vi "Pump Start Detector (Kuhnke) old.vi"(6 "Reset":bool, 9 "Period":i32, 10 "Neg Cross":bool, 11 "Pos Cross":bool) -> (3 "Starts":u32)   [LabVIEW 2019]
uses:
  <vilib>/Platform/TimedLoop/XDataNode/timing_clust.ctl
  <vilib>/Platform/TimedLoop/XDataNode/nitl_modes.ctl
  <vilib>/Platform/TimedLoop/XDataNode/wakeup.ctl
  <vilib>/Platform/TimedLoop/XDataNode/XDataNode.xnode
  <vilib>/Platform/TimedLoop/XDataNode/XDNodeRunTimeDep.lvlib
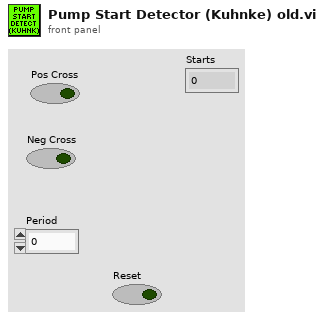
[diagram p1: front panel]
types:
  T1 = typedef "XDNodeRunTimeDep.lvlib/timing_clust.ctl" = cluster{"Expected End [f-1]":u64, "Actual End [f-1]":u64, "Finished Late? [f-1]":bool, "Expected End [i-1]":u64, "Actual End [i-1]":u64, "Finished Late? [i-1]":bool, "Expected Start [i]":u64, "Actual Start [i]":u64, "Expected Start [f]":u64, "Actual Start [f]":u64, "Source Name":string, "Structure Name":string, "Period":i64, "Deadline":i64, "Offset":i64, "Start":i64, "Priority":i32, "Timeout":i32, "Mode":T2, "Wakeup Reason":T3, "Error":errorcluster, "Source Type":string, "Secondary Source Type":string, "Global End Time":u64, "Global Start Time":u64, "Frame Duration":u64, "Iteration Duration":u64, "Assigned CPU":i32, "I/O Scan Engine Mode":u32}
  T2 = typedef "XDNodeRunTimeDep.lvlib/nitl_modes.ctl" = enum32{"No Change", "Process missed periods, maintain original phase", "Discard missed periods, maintain original phase", "Process missed periods, ignore original phase", "Discard missed periods, ignore original phase"}
  T3 = typedef "XDNodeRunTimeDep.lvlib/wakeup.ctl" = enum32{"Normal", "Aborted", "Asynchronous wakeup", "Timing source error", "Timed loop error", "Timeout"}
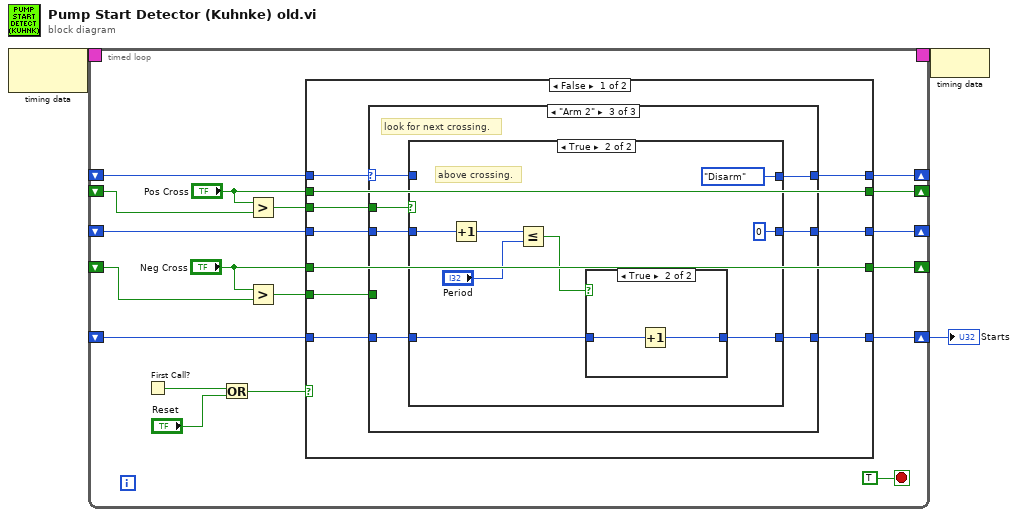
[diagram p0: block diagram]
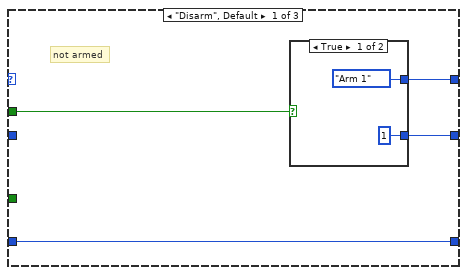
[diagram p2: hidden frame]
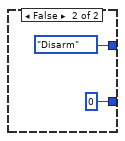
[diagram p3: hidden frame]
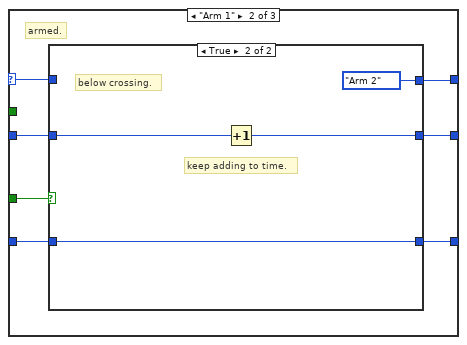
[diagram p4: hidden frame]
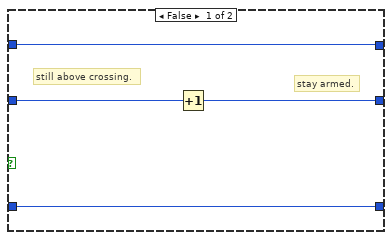
[diagram p5: hidden frame]
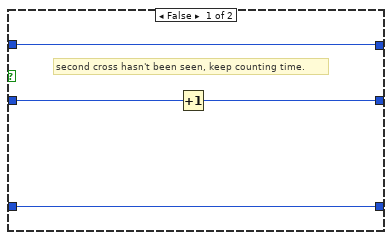
[diagram p6: hidden frame]
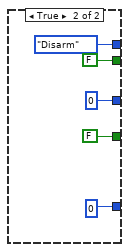
[diagram p8: hidden frame]
diagram:
  n1 = node-c288() -> (w3:T1)  [unwired: 1 in]
  n2 = timed-loop {
    shift-right: [w15] -> w1
    shift-left: _ -> [w16]
    shift-right: [w20] -> _
    shift-left: _ -> [w21]
    shift-right: [w19] -> _
    shift-left: _ -> [w18]
    timing: w3 -> [_]
    timing-out: [_] -> w2
    shift-right: [w12] -> _
    shift-left: _ -> [w10]
    shift-right: [w7] -> _
    shift-left: _ -> [w5]
    stop <- TRUE stop-if-true
    n3 = First Call?() -> (First Call?: T/F=w14:bool)
    n4 = Or(x=w14, y="Reset") -> (x .or. y?=w13:bool)
    n5 = Greater?(x="Pos Cross", y=w10) -> (0:w11:bool)
    n6 = Greater?(x="Neg Cross", y=w5) -> (0:w4:bool)
    n7 = case shown="False" w13 {
      tunnel: w21 -> [w31 _]
      tunnel: [w30 enum16{"Arm 1", "Arm 2", "Disarm"}."Disarm"] -> w20
      tunnel: [w29 0] -> w19
      tunnel: w18 -> [w28 _]
      tunnel: w16 -> [w27 _]
      tunnel: [w26 u32 0] -> w15
      tunnel: "Pos Cross" -> [w25 _]
      tunnel: [w25 FALSE ("Crossing?")] -> w12
      tunnel: w11 -> [w24 _]
      tunnel: "Neg Cross" -> [w23 _]
      tunnel: [w23 FALSE ("Neg Cross")] -> w7
      tunnel: w4 -> [w22 _]
      frame False {
        n8 = case shown="\"Arm 2\"" w31 {
          selector: w31 -> [_ w41 w55]
          tunnel: [w32 w46 w60] -> w30
          tunnel: [w34 w45 w59] -> w29
          tunnel: w28 -> [_ w44 w58]
          tunnel: w24 -> [w33 _ w61]
          tunnel: w27 -> [w35 w43 w57]
          tunnel: [w35 w42 w56] -> w26
          tunnel: w22 -> [_ w40 _]
          frame "Disarm", Default {
            # "not armed"
            n9 = case shown="True" w33 {
              tunnel: [1 0] -> w34
              tunnel: [enum16{"Arm 1", "Arm 2", "Disarm"}."Arm 1" enum16{"Arm 1", "Arm 2", "Disarm"}."Disarm"] -> w32
              frame True {
              }
              frame False {
              }
            }
          }
          frame "Arm 1" {
            # "armed."
            n10 = case shown="True" w40 {
              tunnel: [w47 enum16{"Arm 1", "Arm 2", "Disarm"}."Arm 2"] -> w46
              tunnel: [w49 w51] -> w45
              tunnel: w44 -> [w50 w52]
              tunnel: w43 -> [w48 w54]
              tunnel: [w48 w54] -> w42
              tunnel: w41 -> [w47 _]
              frame False {
                # "stay armed."
                # "still above crossing."
                n11 = Increment(x=w50) -> (x+1=w49:i32)
              }
              frame True {
                # "keep adding to time."
                # "below crossing."
                n12 = Increment(x=w52) -> (x+1=w51:i32)
              }
            }
          }
          frame "Arm 2" {
            # "look for next crossing."
            n13 = case shown="True" w61 {
              tunnel: [w62 enum16{"Arm 1", "Arm 2", "Disarm"}."Disarm"] -> w60
              tunnel: [w64 0] -> w59
              tunnel: w58 -> [w65 w71]
              tunnel: w57 -> [w63 w70]
              tunnel: [w63 w69] -> w56
              tunnel: w55 -> [w62 _]
              frame False {
                # "second cross hasn't been seen, keep counting time."
                n14 = Increment(x=w65) -> (x+1=w64:i32)
              }
              frame True {
                # "above crossing."
                n15 = Increment(x=w71) -> (x+1=w67:i32)
                n16 = Less Or Equal?(x=w67, y="Period") -> (x <= y?=w68:bool)
                n17 = case shown="True" w68 {
                  tunnel: w70 -> [w74 w76]
                  tunnel: [w74 w75] -> w69
                  frame False {
                  }
                  frame True {
                    n18 = Increment(x=w76) -> (x+1=w75:u32)
                  }
                }
              }
            }
          }
        }
      }
      frame True {
      }
    }
  }
  "Starts" <- w1
  n19 = node-c288(w2) -> ()
